vi "Lickometer-Stop.vi"(7 "Device reference":refnum<vi>, 8 "error in (no error)":errorcluster) -> (0 "error out":errorcluster)   [LabVIEW 2015]
doc: "The lickometer has a semaphore reference; this just releases it.\n\nSo it's not strictly necessary to call this (because it gets taken care of when your main VI stops running), but it's still good practice."
uses:
  Typedefs/Lickometer.ctl
  Rack/Typedefs/OutputRequest refnum.ctl
  Rack/Typedefs/OutputRequest.ctl
  Rack/Typedefs/InputData cluster.ctl
  Rack/Methods/Port drivers/DigitalInput-DataCluster.ctl
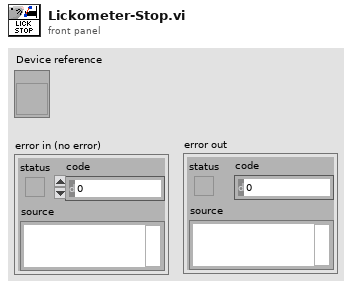
[diagram p1: front panel]
types:
  T1 = typedef "Lickometer.ctl" = cluster{"Settings":cluster{"Min lick duration":u32, "Port name":string, "Port index":i32}, "Lick":bool, "Debouncing":cluster{"Semaphore":T2, "Lick start":u32}, "OutputRequest event ref":T3, "InputData reference":refnum<vi>, "Active hi?":bool}
  T2 = typedef "Semaphore RefNum" = refnum<k1>
  T3 = typedef "OutputRequest refnum.ctl" = refnum<user-event>
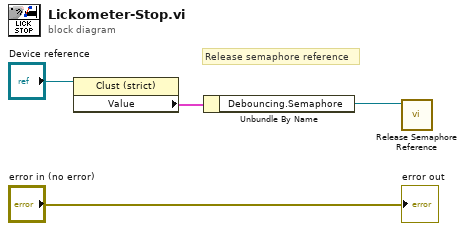
[diagram p0: block diagram]
diagram:
  # "Release semaphore reference"
  n1 = property class="Clust (strict)"(reference="Device reference") -> ("Value"=w3:T1)  [unwired: 1 in, 2 out]
  n2 = Unbundle By Name(w3) -> ("Debouncing.Semaphore"=w2:T2)
  n3 = call <vilib>:"Release Semaphore Reference.vi"("semaphore"=w2) -> ()  [unwired: 9 in, 2 out]
  "error out" <- "error in (no error)"
